vi "2_07.vi"() -> ()   [LabVIEW 2013]
uses:
  <vilib>/Analysis/NI_AALPro.lvlib
  <vilib>/Analysis/2dsp.llb/Upsample (DBL).vi
  <vilib>/Analysis/NI_AALBase.lvlib
  <vilib>/Analysis/3filter.llb/Filter Passband Type.ctl
  <vilib>/Analysis/4window.llb/windowTd.ctl
  <vilib>/Analysis/3filter.llb/FIR Filter (DBL).vi
  <vilib>/Analysis/2dsp.llb/Real FFT.vi
panel:
  out "Comentarios":string="#7.3)  Cantidad de taps 201. Tambien se observa que la frecuencia de transición del filtro ocurre a 60 Hz, 10 Hz mas que la mitad de la frecuencia de muestreo 50 Hz\n\n#7.4)\na) no es posible reconstruir la señal con la frecuencia de muestreo y la cantidad de taps actual\nb) no se elimina por completo la frecuencia imagen \n\n#7.5) Para una señal a 49 Hz con una Fs de 100H, cantidad de taps que se requieren es 4901\n\n#7.6) Una señal cosenoidal a 50Hz si es posible reconstruirse. \nUna señal senoidal a 50Hz  NO se\nreconstruye. Esto puede suceder debido a que no existe una componente impulso positiva y frecuencia positva contenida en la banda pasante del filtro.\nLa frecuencia máxima que es posible reconstruir a 100Hz de tasa de muestreo y con un taps=3500, es 50 Hz.\nA 51Hz la onda reconstruida se desfasa respecto de la original.\n\n#7.7) Con Fs=200Hz, f=49Hz, factor de sobremuestreo=22 y fcorte=100Hz se obtiene una señal similar a la original con un taps=125.\n\nConcluisión: Empleando mayores frecuencias de muestreo, que la establecida por el criterio de Nyquist, se reconstruyen señales mas detalladas y no se requiere de un filtro tan complejo (orden del filtro o taps bajo)"
  in  "Seno":bool
  in  "Frecuencia de corte\nFiltro de reconstruccion":dbl=50.0 format="%0.2f"
  out "Tono y Aliasing\nvs Filtro":waveform(dbl)[](graph)
  in  "Frecuencia de muestreo":dbl=100.0
  out "Muestreo inicial":waveform(dbl)[](graph)
  in  "Cantidad de taps\nFiltro de reconstruccion":i32=1 min=1 step=2
  in  "Factor de sobremuestreo":i32=20
  out "Reconstruccion":waveform(dbl)[](graph)
  in  "Frecuencia de prueba":dbl=10.0
  # "Coseno"
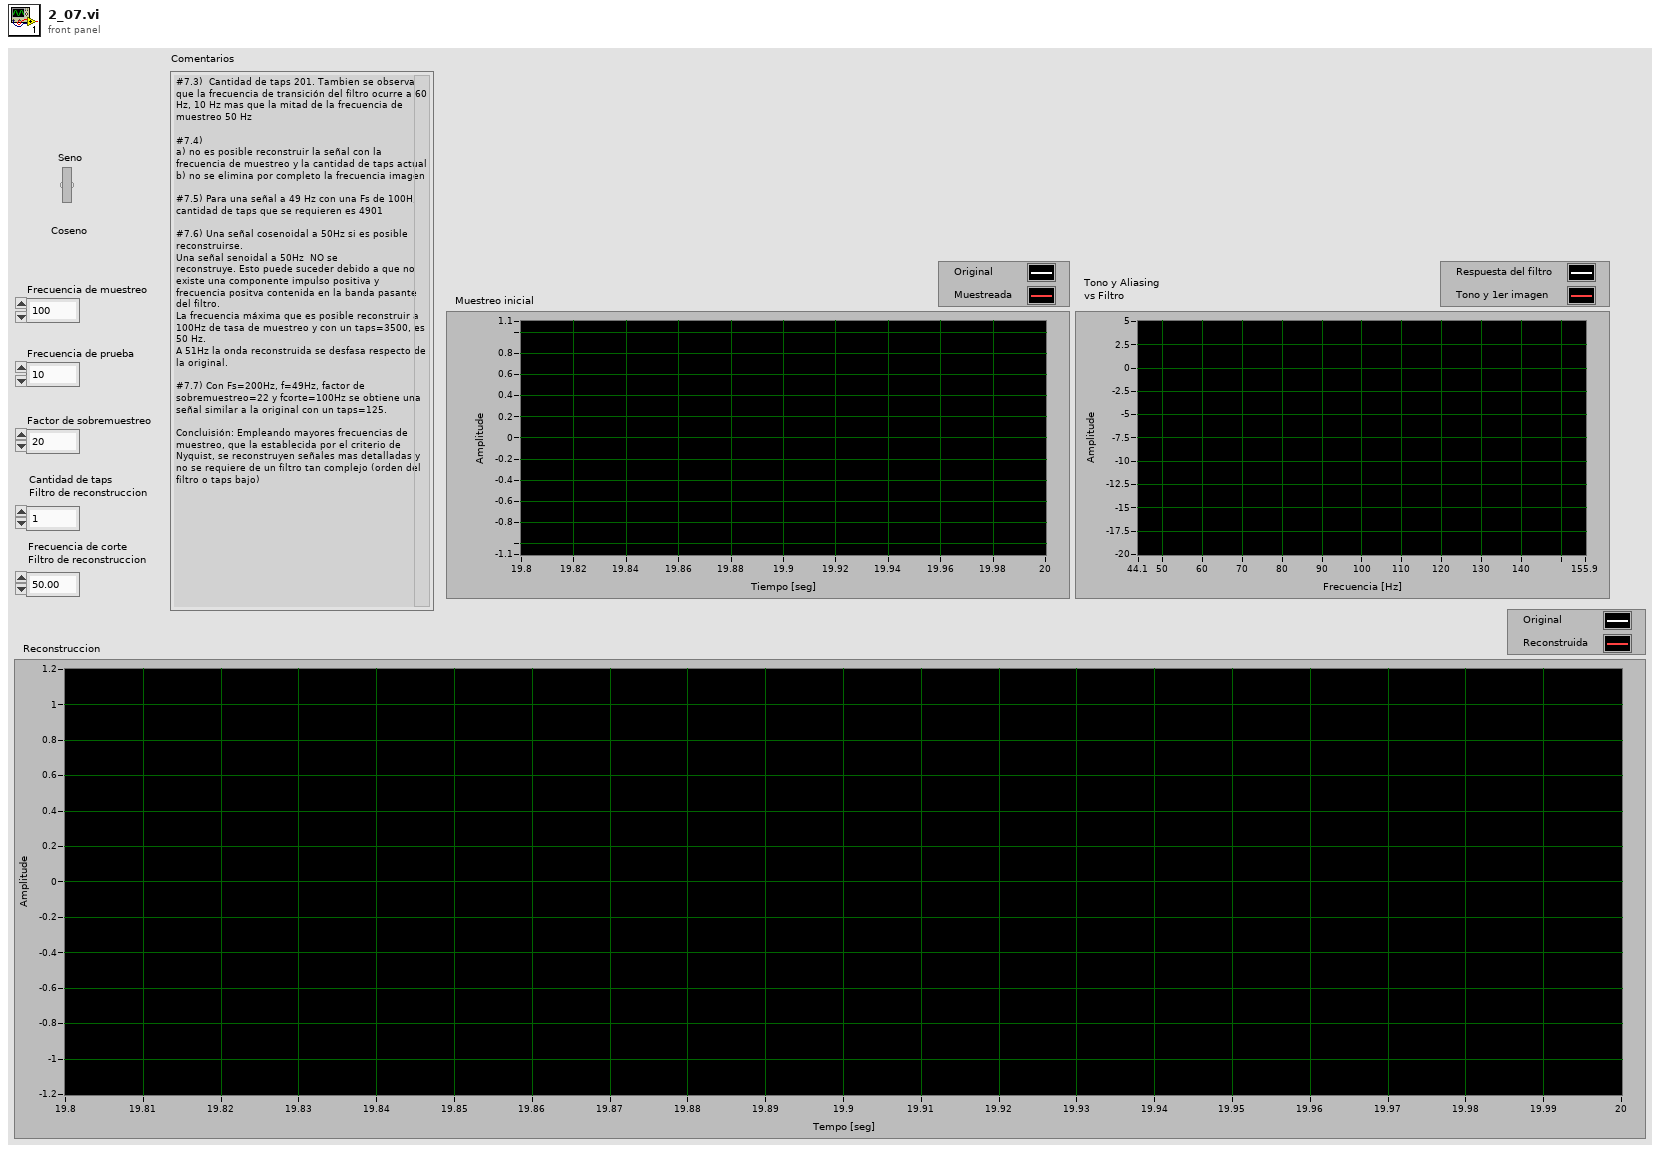
[diagram p1: front panel]
types:
  T1 = typedef "NI_AALPro.lvlib/windowTd.ctl" = u32
  T2 = typedef "NI_AALBase.lvlib/Filter Passband Type.ctl" = enum32{"Lowpass", "Highpass", "Bandpass", "Bandstop"}
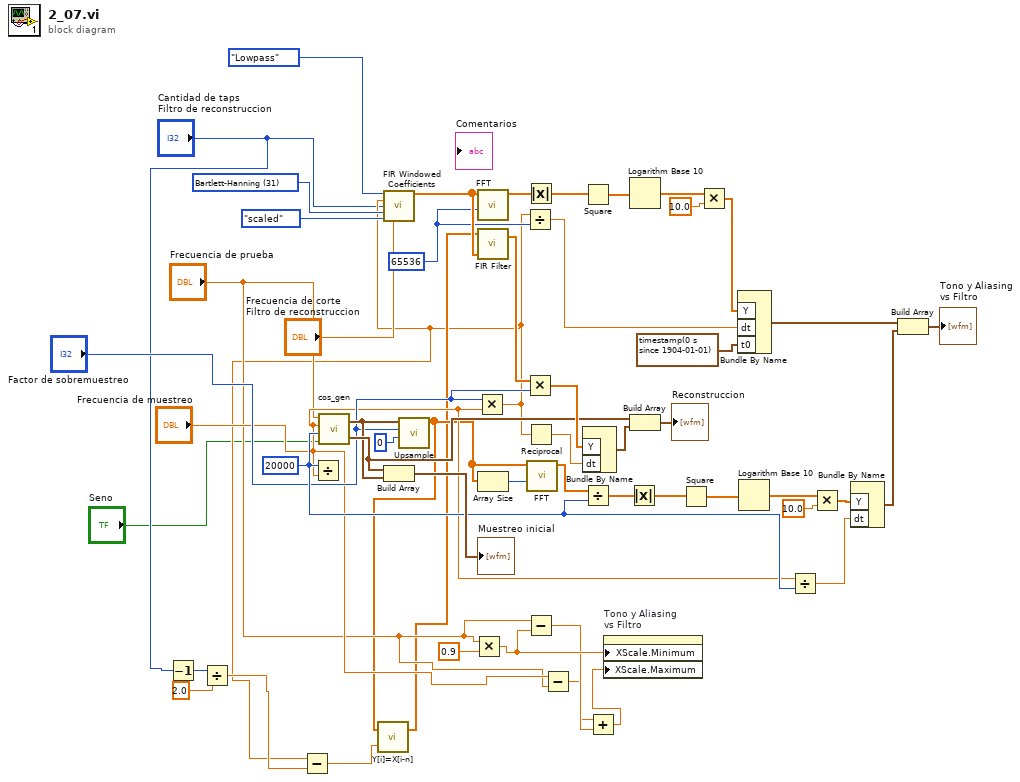
[diagram p0: block diagram]
diagram:
  w24 = 65536 ("FFT size")
  w51 = T1 31 items=["Rectangle"=0, "Hanning"=1, "Hamming"=2, "Blackman-Harris"=3, "Exact Blackman"=4, "Blackman"=5, "Flat Top"=6, "4 Term B-Harris "=7, "7 Term B-Harris"=8, "Low Sidelobe"=9, "Blackman Nuttall"=11, "Triangle"=30, "Bartlett-Hanning"=31, "Bohman"=32, "Parzen"=33, "Welch"=34, "Kaiser"=60, "Dolph-Chebyshev"=61, "Gaussian"=62] ("window")
  w22 = 20000
  n1 = Decrement(x="Cantidad de taps\nFiltro de reconstruccion") -> (x-1=w2:i32)
  n2 = Divide(x=w2, y=2.0) -> (x/y=w6:dbl)
  n3 = Divide(x=w22, y="Frecuencia de muestreo") -> ()  [unwired: 1 out]
  n4 = call "cos_gen.vi"("Seno/Coseno"="Seno", "Cantidad de muestras"=w22, "Frecuencia de muestreo"="Frecuencia de muestreo", "Frecuencia"="Frecuencia de prueba") -> ("Salida Sobremuestreada"=w20:waveform(dbl), "Salida"=w19:waveform(dbl))
  n5 = Build Array(w20, w19) -> (→"Muestreo inicial":waveform(dbl)[])
  n6 = call-poly <vilib>:"Upsample.vi"("leading zeros"=0, "upsampling factor"="Factor de sobremuestreo", "X"=w19) -> ("Upsampled Array"=w9:dbl[])  [unwired: 7 in, 1 out]
  n7 = Multiply(x="Frecuencia de prueba", y=0.9) -> (x*y=w14:dbl)
  n8 = Multiply(x="Factor de sobremuestreo", y="Frecuencia de muestreo") -> (x*y=w5:dbl)
  n9 = Subtract(x=w5, y=w6) -> (x-y=w7:dbl)
  n10 = call <vilib>:"Y[i]=X[i-n].vi"("shifts: n"=w7, "Input Array"=w9) -> ("Shifted Array"=w8:dbl[])  [unwired: 1 out]
  n11 = call <vilib>:"FIR Windowed Coefficients.vi"("filter type"=Filter_Passband_Type."Lowpass", "sampling freq: fs"=w5, "taps"="Cantidad de taps\nFiltro de reconstruccion", "window"=w51, "option"=enum32{"not scaled", "scaled"}."scaled", "low cutoff freq: fl"="Frecuencia de corte\nFiltro de reconstruccion") -> ("FIR Windowed Coefficients"=w45:dbl[])  [unwired: 8 in, 1 out]
  n12 = call-poly <vilib>:"FFT.vi"("FFT size"=w24, "X"=w45) -> ("FFT {X}"=w44:cdb[])  [unwired: 8 in, 1 out]
  n13 = call-poly <vilib>:"FIR Filter.vi"("FIR Coefficients"=w45, "X"=w8) -> ("Filtered X"=w25:dbl[])  [unwired: 2 in, 1 out]
  n14 = Array Size(array=w9) -> (size(s)=w37:i32)
  n15 = Divide(x=w5, y=w24) -> (x/y=w39:dbl)
  n16 = Multiply(x=w25, y="Factor de sobremuestreo") -> (x*y=w48:dbl[])
  n17 = Absolute Value(x=w44) -> (abs(x)=w43:dbl[])
  n18 = Reciprocal(x=w5) -> (1/x=w21:dbl)
  n19 = Subtract(x="Frecuencia de prueba", y=w14) -> (x-y=w12:dbl)
  n20 = call-poly <vilib>:"FFT.vi"("FFT size"=w37, "X"=w9) -> ("FFT {X}"=w32:cdb[])  [unwired: 8 in, 1 out]
  n21 = Subtract(x="Frecuencia de muestreo", y="Frecuencia de prueba") -> (x-y=w11:dbl)
  n22 = Square(x=w43) -> (x^2=w42:dbl[])
  n23 = Bundle By Name("Y"=w48, "dt"=w21) -> (w49:waveform(dbl))  [unwired: 1 in]
  n24 = Divide(x=w32, y=w22) -> (x/y=w27:cdb[])
  n25 = Add(x=w11, y=w12) -> (x+y=w10:dbl)
  n26 = property on="Tono y Aliasing\nvs Filtro" class="WFGraph (strict)"("XScale.Minimum"=w14, "XScale.Maximum"=w10) -> ()  [unwired: 2 in, 2 out]
  n27 = Absolute Value(x=w27) -> (abs(x)=w28:dbl[])
  n28 = Logarithm Base 10(1:w42) -> (0:w40:dbl[])
  n29 = Build Array(w20, w49) -> (→"Reconstruccion":waveform(dbl)[])
  n30 = Square(x=w28) -> (x^2=w29:dbl[])
  n31 = Multiply(x=w40, y=10.0) -> (x*y=w38:dbl[])
  n32 = Bundle By Name("Y"=w38, "dt"=w39, "t0"=timestamp(0 s since 1904-01-01)) -> (w35:waveform(dbl))  [unwired: 1 in]
  n33 = Logarithm Base 10(1:w29) -> (0:w31:dbl[])
  n34 = Divide(x="Frecuencia de muestreo", y=w22) -> (x/y=w23:dbl)
  n35 = Multiply(x=w31, y=10.0) -> (x*y=w26:dbl[])
  n36 = Bundle By Name("Y"=w26, "dt"=w23) -> (w34:waveform(dbl))  [unwired: 1 in]
  n37 = Build Array(w35, w34) -> (→"Tono y Aliasing\nvs Filtro":waveform(dbl)[])
